vi "TCP Read sobot Commands.vi"(8 "error in (no error)":errorcluster, 11 "TCP Network Connection in":refnum<k5>) -> (0 "error out":errorcluster, 1 "SoBot_CommandTypes":T1, 2 "data out":string, 3 "TCP Network Connection out":refnum<k5>)   [LabVIEW 2017]
uses:
  sobot structures/SoBot_CommandTypes.ctl
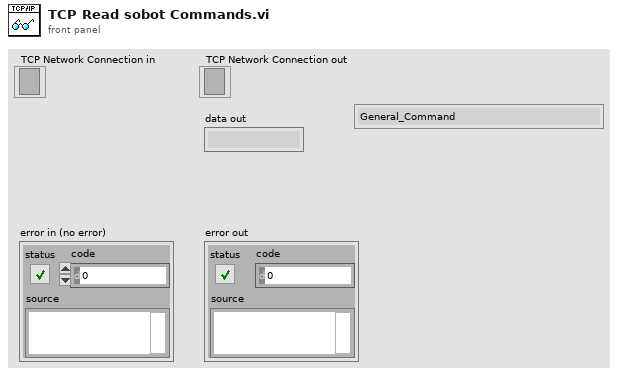
[diagram p1: front panel]
types:
  T1 = typedef "SoBot_CommandTypes.ctl" = enum16{"General_Command", "XY_Command", "Z_Command", "Plattform_Command"}
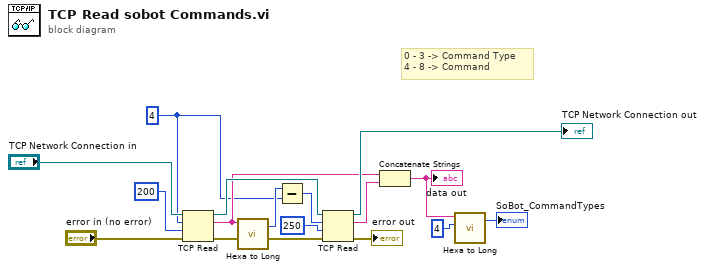
[diagram p0: block diagram]
diagram:
  w1 = 4 ("bytes to read")
  # "0 - 3 -> Command Type\n4 - 8 -> Command"
  n1 = TCP Read(connection ID="TCP Network Connection in", bytes to read=w1, error in (no error)="error in (no error)", 9:200 ("timeout ms (25000)")) -> (connection ID out=w14:refnum<k5>, data out=w5:string, error out=w13:errorcluster)  [unwired: 1 in]
  n2 = call "Hexa to Long.vi"("Hexa"=w5) -> ("Long"=w8:u32)  [unwired: 5 in]
  n3 = Subtract(x=w8, y=w1) -> (x-y=w7:u32)
  n4 = TCP Read(connection ID=w14, bytes to read=w7, error in (no error)=w13, 9:250 ("timeout ms (25000)")) -> (connection ID out=→"TCP Network Connection out":refnum<k5>, data out=w6:string, error out=→"error out":errorcluster)  [unwired: 1 in]
  n5 = Concatenate Strings(w5, w6) -> (w4:string)
  "data out" <- w4
  n6 = call "Hexa to Long.vi"("Hexa"=w4, "Index"=4) -> ("Long"=→"SoBot_CommandTypes":u32)  [unwired: 4 in]
